vi "Ranges of Center Shoot.vi"(10 "offsetAngle V":dbl, 11 "offsetAngle H":dbl) -> (3 "Boolean":bool)   [LabVIEW 2023]
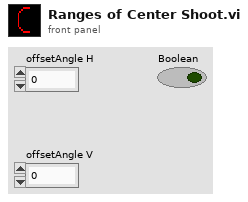
[diagram p1: front panel]
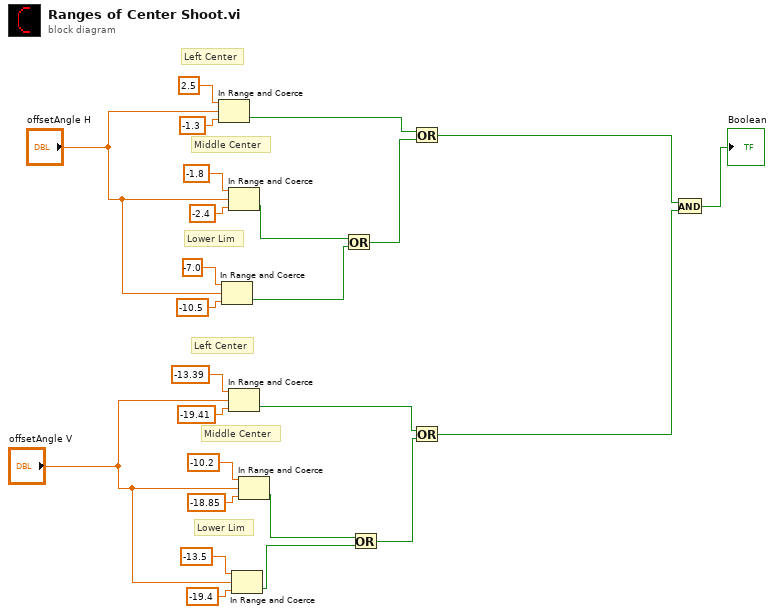
[diagram p0: block diagram]
diagram:
  # "Lower Lim"
  # "Middle Center"
  # "Left Center"
  # "Lower Lim"
  # "Middle Center"
  # "Left Center"
  n1 = In Range and Coerce(upper limit=2.5, x="offsetAngle H", lower limit=-1.3) -> (In Range?=w4:bool)  [unwired: 1 out]
  n2 = In Range and Coerce(upper limit=-7.0, x="offsetAngle H", lower limit=-10.5) -> (In Range?=w3:bool)  [unwired: 1 out]
  n3 = In Range and Coerce(upper limit=-1.8, x="offsetAngle H", lower limit=-2.4) -> (In Range?=w2:bool)  [unwired: 1 out]
  n4 = In Range and Coerce(upper limit=-13.39, x="offsetAngle V", lower limit=-19.41) -> (In Range?=w8:bool)  [unwired: 1 out]
  n5 = In Range and Coerce(upper limit=-13.5, x="offsetAngle V", lower limit=-19.4) -> (In Range?=w10:bool)  [unwired: 1 out]
  n6 = In Range and Coerce(upper limit=-10.2, x="offsetAngle V", lower limit=-18.85) -> (In Range?=w9:bool)  [unwired: 1 out]
  n7 = Or(x=w2, y=w3) -> (x .or. y?=w5:bool)
  n8 = Or(x=w9, y=w10) -> (x .or. y?=w7:bool)
  n9 = Or(x=w4, y=w5) -> (x .or. y?=w1:bool)
  n10 = Or(x=w8, y=w7) -> (x .or. y?=w6:bool)
  n11 = And(x=w1, y=w6) -> (x .and. y?=→"Boolean":bool)
